vi "Build Types.vi"(7 "Output Folder":path, 8 "error in (no error)":errorcluster, 9 "Messages":map{string, T3}(c390), 10 "Enumerations":map{string, T1}(c390), 11 "LV-Protoc in":refnum<class "LV-Protoc.lvclass">) -> (0 "error out":errorcluster, 3 "LV-Protoc out":refnum<class "LV-Protoc.lvclass">)   [LabVIEW 2020, in "LV-Protoc.lvlib" / "LV-Protoc.lvclass"]
uses:
  LV-Protoc.lvclass
  LV-Proto/Message.ctl
  LV-Proto/Field.ctl
  LV-Proto/Type.ctl
  LV-Proto/Proto Type.ctl
  LV-Proto/Enumeration.ctl
  LV-Proto/Enum Value.ctl
  LV-Protoc.lvclass/LV-Protoc.ctl
  LV-Protoc.lvlib
  LV-Proto/LV-Proto.lvlib
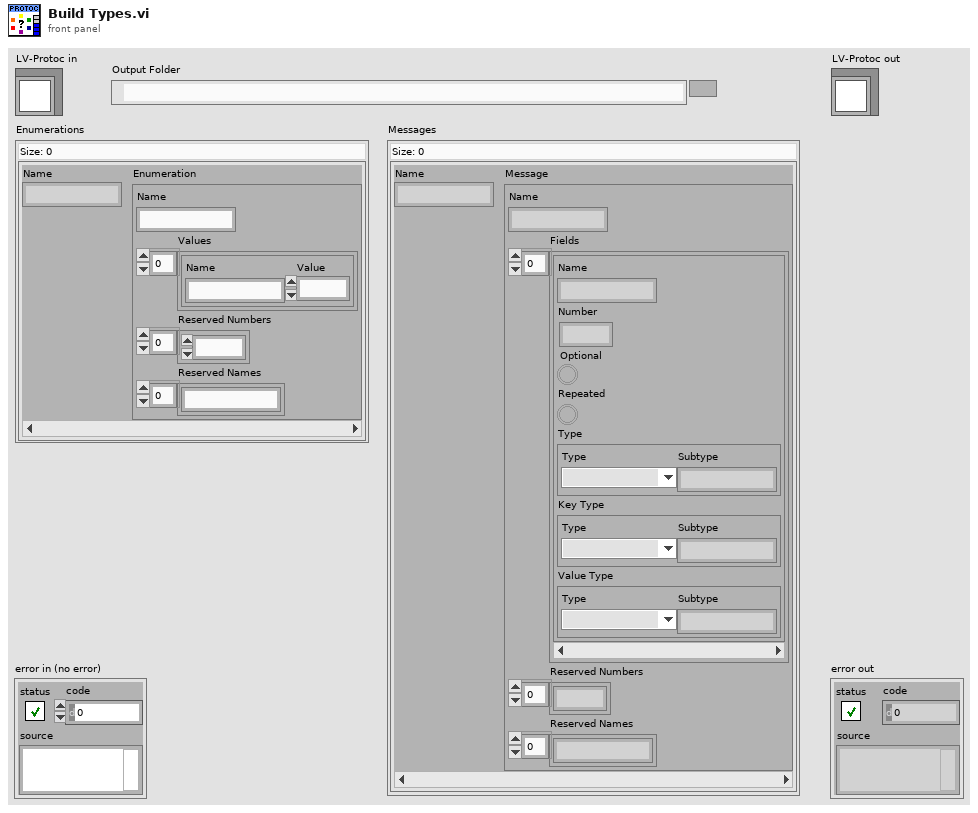
[diagram p1: front panel]
types:
  T1 = typedef "LV-Proto.lvlib/Enumeration.ctl" = cluster{"Name":string, "Values":T2[], "Reserved Numbers":u32[], "Reserved Names":string[]}
  T2 = typedef "LV-Proto.lvlib/Enum Value.ctl" = cluster{"Name":string, "Value":i32}
  T3 = typedef "LV-Proto.lvlib/Message.ctl" = cluster{"Name":string, "Fields":T4[], "Reserved Numbers":u32[], "Reserved Names":string[]}
  T4 = typedef "LV-Proto.lvlib/Field.ctl" = cluster{"Name":string, "Number":u32, "Optional":bool, "Repeated":bool, "Type":T5, "Key Type":T5, "Value Type":T5}
  T5 = typedef "LV-Proto.lvlib/Type.ctl" = cluster{"Type":T6, "Subtype":string}
  T6 = typedef "LV-Proto.lvlib/Proto Type.ctl" = enum16{"UNKNOWN", "double", "float", "int32", "int64", "uint32", "uint64", "sint32", "sint64", "fixed32", "fixed64", "sfixed32", "sfixed64", "bool", "string", "bytes", "enum", "map", "message"}
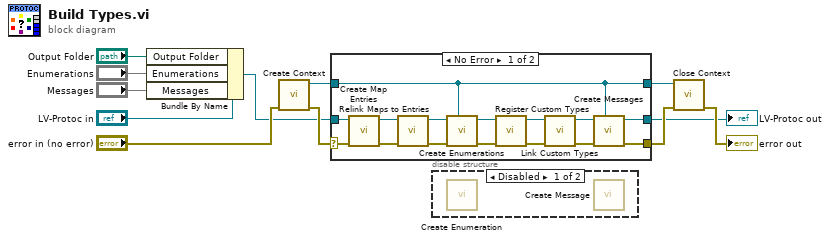
[diagram p0: block diagram]
diagram:
  n1 = Bundle By Name(cluster="LV-Protoc in", "Output Folder"="Output Folder", "Enumerations"="Enumerations", "Messages"="Messages") -> (w4:refnum<class "LV-Protoc.lvclass">)
  n2 = call "Create Context.vi"("error in (no error)"="error in (no error)") -> ("error out"=w10:errorcluster, "App"=w2:refnum<vi>)  [unwired: 9 in]
  n3 = case shown="No Error" w10 {
    selector: w10 -> [w14 w29]
    tunnel: w4 -> [w27 w30]
    tunnel: [w21 w29] -> w12
    tunnel: [w20 w30] -> w3
    tunnel: w2 -> [w13 w28]
    tunnel: [w13 w28] -> w1
    frame No Error {
      n4 = call "Create Map Entries.vi"("error in (no error)"=w14, "LV-Protoc in"=w27) -> ("error out"=w25:errorcluster, "LV-Protoc out"=w26:refnum<class "LV-Protoc.lvclass">)  [unwired: 8 in]
      n5 = call "Relink Maps to Entries.vi"("error in (no error)"=w25, "LV-Protoc in"=w26) -> ("error out"=w24:errorcluster, "LV-Protoc out"=w22:refnum<class "LV-Protoc.lvclass">)  [unwired: 8 in]
      n6 = call "Create Enumerations.vi"("App"=w13, "error in (no error)"=w24, "LV-Protoc in"=w22) -> ("error out"=w23:errorcluster, "LV-Protoc out"=w18:refnum<class "LV-Protoc.lvclass">)  [unwired: 7 in]
      n7 = call "Register Custom Types.vi"("error in (no error)"=w23, "LV-Protoc in"=w18) -> ("error out"=w19:errorcluster, "LV-Protoc out"=w16:refnum<class "LV-Protoc.lvclass">)  [unwired: 8 in]
      n8 = call "Link Custom Types.vi"("error in (no error)"=w19, "LV-Protoc in"=w16) -> ("error out"=w17:errorcluster, "LV-Protoc out"=w15:refnum<class "LV-Protoc.lvclass">)  [unwired: 8 in]
      n9 = call "Create Messages.vi"("App"=w13, "error in (no error)"=w17, "LV-Protoc in"=w15) -> ("error out"=w21:errorcluster, "LV-Protoc out"=w20:refnum<class "LV-Protoc.lvclass">)  [unwired: 7 in]
    }
    frame Error {
    }
  }
  "LV-Protoc out" <- w3
  n10 = disable-structure shown="Disabled" {
    frame Disabled {
      n11 = call "Create Enumeration.vi"() -> ()  [unwired: 10 in, 2 out]
      n12 = call "Create Message.vi"() -> ()  [unwired: 9 in, 3 out]
    }
    frame Enabled {
    }
  }
  n13 = call "Close Context.vi"("error in (no error)"=w12, "App"=w1) -> ("error out"=→"error out":errorcluster)  [unwired: 9 in]
